vi "Read Wavenames.vi"(8 "error in (no error)":errorcluster, 11 "Data Save":refnum<class "LV-Data.lvclass">) -> (0 "error out":errorcluster, 2 "Wavenames":string[](array[string]), 3 "Data Save out":refnum<class "LV-Data.lvclass">)   [LabVIEW 2019, in "LV-Data.lvclass"]
uses:
  LV-Data.lvclass
  LV-Data.lvclass/LV-Data.ctl
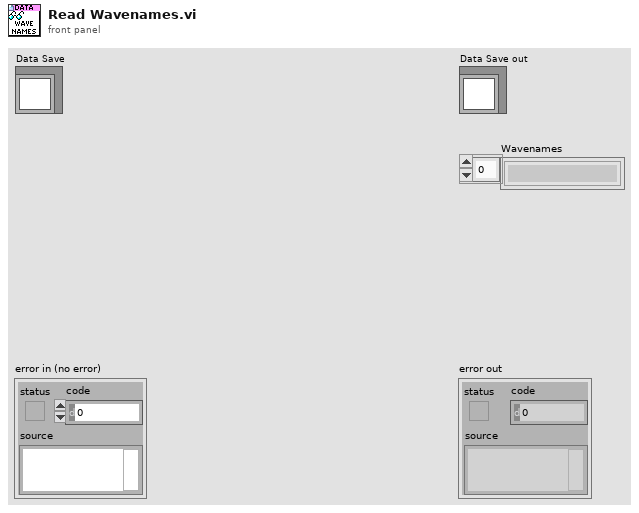
[diagram p1: front panel]
types:
  T1 = typedef "LV-Data.lvclass/Dictionary--cluster.ctl" = cluster{"key":string, "value":variant}
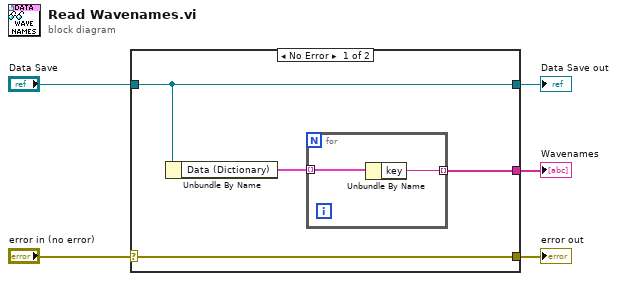
[diagram p0: block diagram]
diagram:
  n1 = case shown="No Error" "error in (no error)" {
    selector: "error in (no error)" -> [w9 w12]
    tunnel: [w9 w12] -> w4
    tunnel: [w8 w13] -> w2
    tunnel: "Data Save" -> [w8 w13]
    tunnel: [w6 _] -> w1
    frame No Error {
      n2 = Unbundle By Name(w8) -> ("Data (Dictionary)"=w7:T1[])
      n3 = for {
        tunnel: w7 -> [w11] mode=indexing
        tunnel: [w10] -> w6 mode=indexing
        n4 = Unbundle By Name(w11) -> ("key"=w10:string)
      }
    }
    frame Error {
    }
  }
  "error out" <- w4
  "Data Save out" <- w2
  "Wavenames" <- w1
